vi "Configure Coupling.vi"(6 "Enable Coupling (T: Enable)":bool=TRUE, 7 "Deviation (0)":dbl, 8 "error in (no error)":errorcluster, 9 "Enable Track (F: Disable)":bool, 10 "Action Type (0: Set Amplitude Coupling)":i32(ring) items=["Set Amplitude Coupling", "Set Frequency Coupling", "Set Phase Coupling"], 11 "VISA resource name":refnum<visa-resource-name>) -> (0 "error out":errorcluster, 3 "VISA resource name out":refnum<visa-resource-name>)   [LabVIEW 2015, in "SDG X Series.lvlib"]
doc: "Configures the coupling settings."
uses:
  <instrlib>/SDG X Series/SDG X Series.lvlib
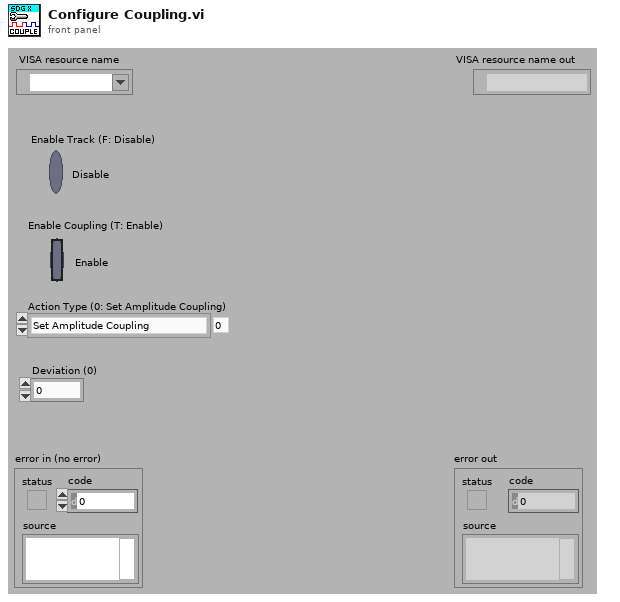
[diagram p1: front panel]
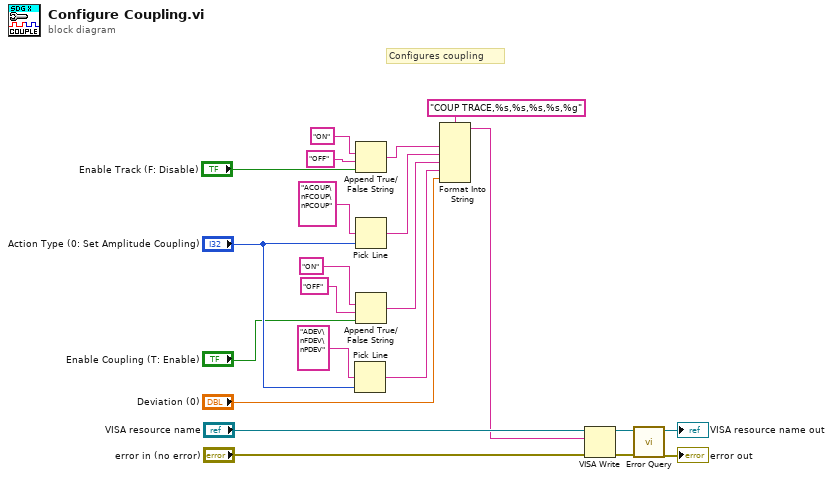
[diagram p0: block diagram]
diagram:
  # "Configures coupling"
  n1 = Pick Line(multi-line string="ADEV\nFDEV\nPDEV", line index="Action Type (0: Set Amplitude Coupling)") -> (output string=w3:string)  [unwired: 1 out]
  n2 = Append True/False String(1:"Enable Track (F: Disable)", 2:"OFF", 3:"ON") -> (0:w6:string)  [unwired: 1 out]
  n3 = Pick Line(multi-line string="ACOUP\nFCOUP\nPCOUP", line index="Action Type (0: Set Amplitude Coupling)") -> (output string=w5:string)  [unwired: 1 out]
  n4 = Append True/False String(1:"Enable Coupling (T: Enable)", 2:"OFF", 3:"ON") -> (0:w4:string)  [unwired: 1 out]
  n5 = Format Into String(format string="COUP TRACE,%s,%s,%s,%s,%g", w6, w5, w4, w3, "Deviation (0)") -> (resulting string=w9:string)  [unwired: 2 in, 1 out]
  n6 = VISA Write(VISA resource name="VISA resource name", write buffer=w9, error in (no error)="error in (no error)") -> (VISA resource name out=w20:refnum<visa-resource-name>, error out=w19:errorcluster)  [unwired: 1 out]
  n7 = call <instrlib>:"Error Query.vi"("error in (no error)"=w19, "VISA resource name"=w20) -> ("error out"=→"error out":errorcluster, "VISA resource name out"=→"VISA resource name out":refnum<visa-resource-name>)  [unwired: 6 in, 2 out]
